vi "Error Query.vi"(8 "error in (no error)":errorcluster, 11 "VISA resource name":refnum<visa-resource-name>) -> (0 "error out":errorcluster, 2 "Error Message":string, 3 "VISA resource name out":refnum<visa-resource-name>)   [LabVIEW 2019, in "Lake Shore 325.lvlib"]
doc: "Queries the instrument for any errors or warnings in the instrument's status system.\n\nThe following conditions will be returned as errors in the Error Out cluster:\n<B>Processor Communication Error</B>\n<B>Query Error</B>\n<B>Execution Error</B>\n<B>Command Error</B>\n\nThe following conditions will be returned as warnings in the Error Out cluster:\n<B>Sensor A Overload</B>\n<B>Sensor B Overload</B>\n\nNote:\nThis VI is called automatically by most driver VIs so it is not usually necessary to call this in an application."
uses:
  <instrlib>/Lake Shore 325/Lake Shore 325.lvlib
  Instance           3 19Saved   Error Query .vi
  Instance           4 19Saved   Error Query .vi
  Instance           2 19Saved   Error Query .vi
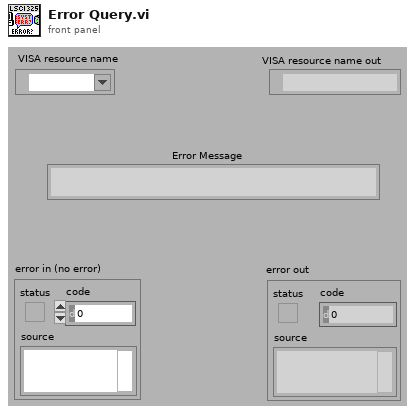
[diagram p1: front panel]
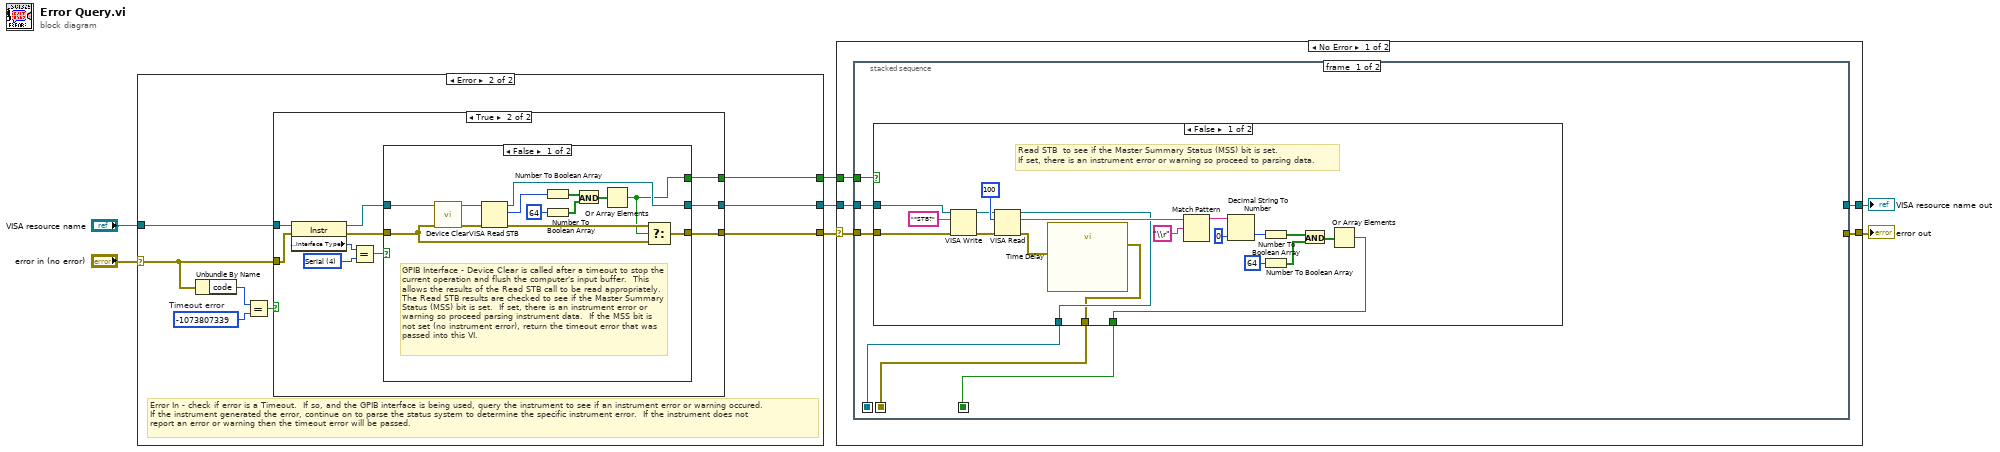
[diagram p0: block diagram]
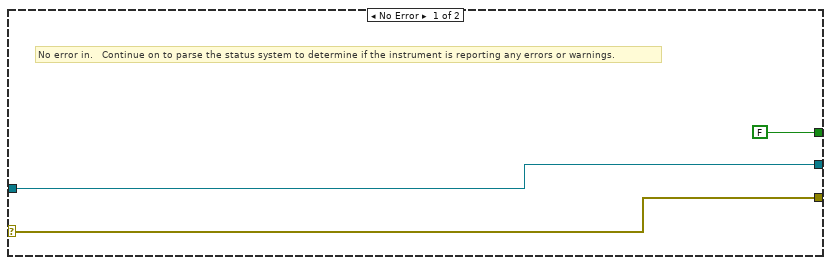
[diagram p2: hidden frame]
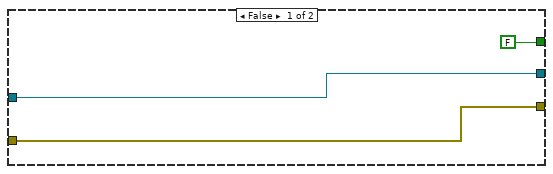
[diagram p3: hidden frame]
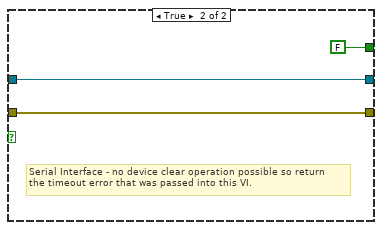
[diagram p4: hidden frame]
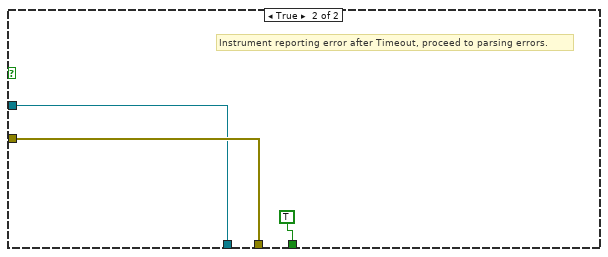
[diagram p5: hidden frame]
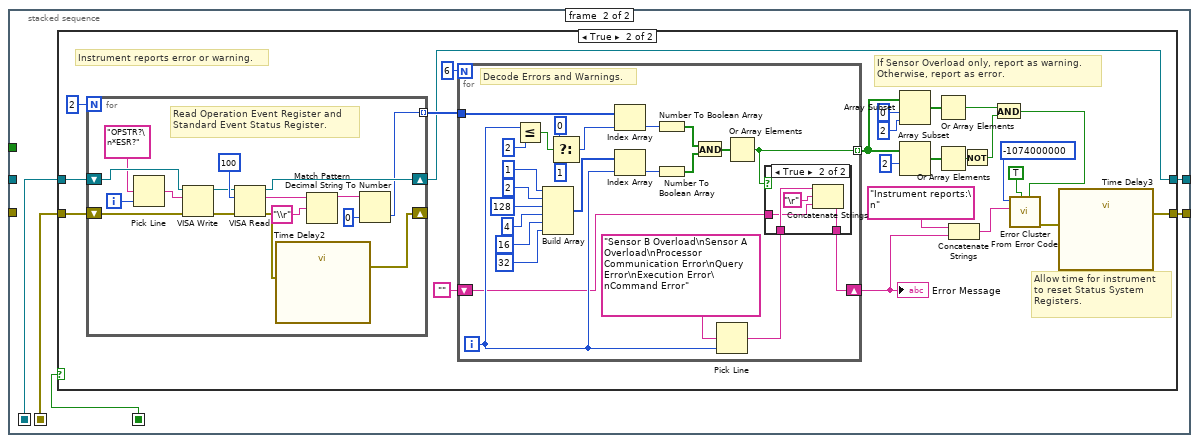
[diagram p6: hidden frame]
diagram:
  n1 = case shown="Error" "error in (no error)" {
    selector: "error in (no error)" -> [w10 w14]
    tunnel: "VISA resource name" -> [w9 w15]
    tunnel: [w10 w13] -> w5
    tunnel: [w9 w12] -> w4
    tunnel: [FALSE w11] -> w3
    frame No Error {
      # "No error in.   Continue on to parse the status system to determine if the instrument is reporting any errors or warnings."
    }
    frame Error {
      w17 = -1073807339  # Timeout error
      # "Error In - check if error is a Timeout.  If so, and the GPIB interface is being used, query the instrument to see if an instrument error or warning occured.  \nIf the instrument generated the error, continue on to parse the status system to determine the specific instrument error.  If the instrument does not \nreport an error or warning then the timeout error will be passed."
      n2 = Unbundle By Name(w14) -> ("code"=w18:i32)
      n3 = Equal?(x=w18, y=w17) -> (x = y?=w16:bool)
      n4 = case shown="True" w16 {
        tunnel: w15 -> [w20 w30]
        tunnel: w14 -> [w21 w29]
        tunnel: [w21 w25] -> w13
        tunnel: [w20 w23] -> w12
        tunnel: [FALSE w22] -> w11
        frame False {
        }
        frame True {
          w28 = u16 4 items=["GPIB"=1, "VXI"=2, "GPIB-VXI"=3, "Serial"=4, "PXI"=5, "TCPIP"=6, "USB"=7] ("Interface Information:Interface Type")
          n5 = property class="Instr"(reference=w30, error in=w29) -> (reference out=w24:refnum<visa-resource-name>, error out=w26:errorcluster, "Interface Information:Interface Type"=w31:u16)
          n6 = Equal?(x=w31, y=w28) -> (x = y?=w27:bool)
          n7 = case shown="False" w27 {
            tunnel: w26 -> [w34 w45]
            tunnel: [w35 w45] -> w25
            tunnel: w24 -> [w39 w46]
            tunnel: [w36 w46] -> w23
            tunnel: [w33 FALSE] -> w22
            frame False {
              # "GPIB Interface - Device Clear is called after a timeout to stop the current operation and flush the computer's input buffer.  This allows the results of the Read STB call to be read appropriately.  The Read STB results are checked to see if the Master Summary Status (MSS) bit is set.  If set, there is an instrument error or warning so proceed parsing instrument data.  If the MSS bit is not set (no instrument error), return the timeout error that was passed into this VI."
              n8 = call <instrlib>:"Device Clear.vi"("error in (no error)"=w34, "VISA Resource Name"=w39) -> ("error out"=w38:errorcluster, "VISA Resource Out"=w37:refnum<visa-resource-name>)  [unwired: 8 in]
              n9 = VISA Read STB(8:w38, 11:w37) -> (0:w40:errorcluster, 2:w32:u16, 3:w36:refnum<visa-resource-name>)
              n10 = Number To Boolean Array(number=w32) -> (Boolean array=w41:bool[])
              n11 = Number To Boolean Array(number=64) -> (Boolean array=w43:bool[])
              n12 = And(x=w41, y=w43) -> (x .and. y?=w42:bool[])
              n13 = Or Array Elements(Boolean array=w42) -> (logical OR=w33:bool)
              n14 = Select(t=w40, s=w33, f=w34) -> (s? t:f=w35:errorcluster)
            }
            frame True {
              # "Serial Interface - no device clear operation possible so return \nthe timeout error that was passed into this VI."
            }
          }
        }
      }
    }
  }
  n15 = case shown="No Error" w5 {
    selector: w5 -> [w50 w158]
    tunnel: w4 -> [w51 w157]
    tunnel: w3 -> [w52 _]
    tunnel: [w49 w158] -> w1
    tunnel: [w48 w157] -> w2
    frame No Error {
      n16 = stacked-sequence {
        seq-local: [w55 _] -> [_ w81]
        seq-local: [w54 _] -> [_ w85]
        seq-local: [w53 _] -> [_ w84]
        tunnel: w52 -> [w58 _]
        tunnel: w51 -> [w57 _]
        tunnel: w50 -> [w56 _]
        tunnel: [_ w83] -> w48
        tunnel: [_ w82] -> w49
        frame #0 {
          n17 = case shown="False" w58 {
            tunnel: w57 -> [w60 w79]
            tunnel: w56 -> [w59 w80]
            tunnel: [w65 TRUE] -> w55
            tunnel: [w61 w80] -> w53
            tunnel: [w64 w79] -> w54
            frame False {
              # "Read STB  to see if the Master Summary Status (MSS) bit is set.\nIf set, there is an instrument error or warning so proceed to parsing data."
              n18 = VISA Write(VISA resource name=w60, write buffer="*STB?", error in (no error)=w59) -> (VISA resource name out=w75:refnum<visa-resource-name>, error out=w74:errorcluster)  [unwired: 1 out]
              n19 = VISA Read(VISA resource name=w75, byte count=100, error in (no error)=w74) -> (VISA resource name out=w64:refnum<visa-resource-name>, read buffer=w77:string, error out=w62:errorcluster)  [unwired: 1 out]
              n20 = call "Time Delay"("error in (no error)"=w62) -> ("error out"=w61:errorcluster)  [unwired: 10 in]
              n21 = Match Pattern(string=w77, regular expression="\\r") -> (before substring=w70:string)  [unwired: 1 in, 3 out]
              n22 = Decimal String To Number(string=w70, default (0L)=u16 0) -> (number=w63:u16)  [unwired: 1 in, 1 out]
              n23 = Number To Boolean Array(number=w63) -> (Boolean array=w66:bool[])
              n24 = Number To Boolean Array(number=64) -> (Boolean array=w68:bool[])
              n25 = And(x=w66, y=w68) -> (x .and. y?=w67:bool[])
              n26 = Or Array Elements(Boolean array=w67) -> (logical OR=w65:bool)
            }
            frame True {
              # "Instrument reporting error after Timeout, proceed to parsing errors."
            }
          }
        }
        frame #1 {
          n27 = case shown="True" w81 {
            tunnel: w85 -> [w87 w110]
            tunnel: w84 -> [w86 w109]
            tunnel: [w87 w105] -> w83
            tunnel: [w86 w90] -> w82
            frame False {
              # "No instrument error or warning reported."
            }
            frame True {
              # "Allow time for instrument\nto reset Status System\nRegisters."
              # "If Sensor Overload only, report as warning.\nOtherwise, report as error."
              # "Instrument reports error or warning."
              n28 = for {
                N: 2 -> [_]
                shift-right: [w154] -> w105
                shift-left: w110 -> [w155]
                shift-right: [w141] -> _
                shift-left: w109 -> [w143]
                tunnel: [w144] -> w106 mode=indexing
                i -> [w156]
                # "Read Operation Event Register and \nStandard Event Status Register."
                n29 = Pick Line(multi-line string="OPSTR?\n*ESR?", line index=w156) -> (output string=w145:string)  [unwired: 1 in]
                n30 = VISA Write(VISA resource name=w155, write buffer=w145, error in (no error)=w143) -> (VISA resource name out=w151:refnum<visa-resource-name>, error out=w150:errorcluster)  [unwired: 1 out]
                n31 = VISA Read(VISA resource name=w151, byte count=100, error in (no error)=w150) -> (VISA resource name out=w154:refnum<visa-resource-name>, read buffer=w153:string, error out=w142:errorcluster)  [unwired: 1 out]
                n32 = call "Time Delay2"("error in (no error)"=w142) -> ("error out"=w141:errorcluster)  [unwired: 10 in]
                n33 = Match Pattern(string=w153, regular expression="\\r") -> (before substring=w147:string)  [unwired: 1 in, 3 out]
                n34 = Decimal String To Number(string=w147, default (0L)=u16 0) -> (number=w144:u16)  [unwired: 1 in, 1 out]
              }
              n35 = for {
                N: 6 -> [_]
                shift-right: [w116] -> w103
                shift-left: "" -> [w118]
                tunnel: w106 -> [w128]
                tunnel: [w119] -> w98 mode=indexing
                i -> [w122]
                # "Decode Errors and Warnings."
                n36 = Less Or Equal?(x=w122, y=2) -> (x <= y?=w127:bool)
                n37 = Build Array(1, 2, 128, 4, 16, 32) -> (w132:i32[])
                n38 = Select(t=0, s=w127, f=1) -> (s? t:f=w124:i32)
                n39 = Index Array(array=w128, index=w124) -> (element=w123:u16)
                n40 = Index Array(array=w132, index=w122) -> (element=w131:i32)
                n41 = Number To Boolean Array(number=w123) -> (Boolean array=w133:bool[])
                n42 = Number To Boolean Array(number=w131) -> (Boolean array=w135:bool[])
                n43 = And(x=w133, y=w135) -> (x .and. y?=w134:bool[])
                n44 = Pick Line(multi-line string="Sensor B Overload\nSensor A Overload\nProcessor Communication Error\nQuery Error\nExecution Error\nCommand Error", line index=w122) -> (output string=w117:string)  [unwired: 1 in]
                n45 = Or Array Elements(Boolean array=w134) -> (logical OR=w119:bool)
                n46 = case shown="True" w119 {
                  tunnel: w118 -> [w136 w137]
                  tunnel: w117 -> [_ w140]
                  tunnel: [w136 w139] -> w116
                  frame False {
                  }
                  frame True {
                    n47 = Concatenate Strings(w140, "\r", w137) -> (w139:string)
                  }
                }
              }
              "Error Message" <- w103
              n48 = Array Subset(array=w98, index=0, length=2) -> (w96:bool[])
              n49 = Array Subset(array=w98, index=2) -> (w95:bool[])  [unwired: 1 in]
              n50 = Or Array Elements(Boolean array=w96) -> (logical OR=w94:bool)
              n51 = Or Array Elements(Boolean array=w95) -> (logical OR=w93:bool)
              n52 = Concatenate Strings("Instrument reports:\n" ("Source"), w103) -> (w100:string)
              n53 = Not(x=w93) -> (.not. x?=w92:bool)
              n54 = And(x=w94, y=w92) -> (x .and. y?=w88:bool)
              n55 = call <vilib>:"Error Cluster From Error Code.vi"("is warning? (False)"=w88, "show call chain? (False)"=TRUE, "error message (\"\")"=w100, "error code (0)"=-1074000000 ("Code")) -> ("error out"=w89:errorcluster)  [unwired: 5 in]
              n56 = call "Time Delay3"("error in (no error)"=w89) -> ("error out"=w90:errorcluster)  [unwired: 10 in]
            }
          }
        }
      }
    }
    frame Error {
    }
  }
  "error out" <- w1
  "VISA resource name out" <- w2
